vi "BAM Buffer Connections List.vi"(7 "State":T2=enum."Update", 8 "error in (no error)":errorcluster, 9 "index":i32, 10 "Connection Cluster":T3, 11 "Connections Ref":T1) -> (0 "error out":errorcluster, 1 "Connections":T3[](array[typedef]), 2 "Connection Cluster Out":T3, 3 "Connections Ref out":T1)   [LabVIEW 2015, in "J1939 Addon Engine.lvlib"]
uses:
  J1939 Addon Engine.lvlib
  Types/TP Buffer Connection Cluster.ctl
  Types/TP Connections List State.ctl
  Types/BAM Buffer Connections List_Ref.ctl
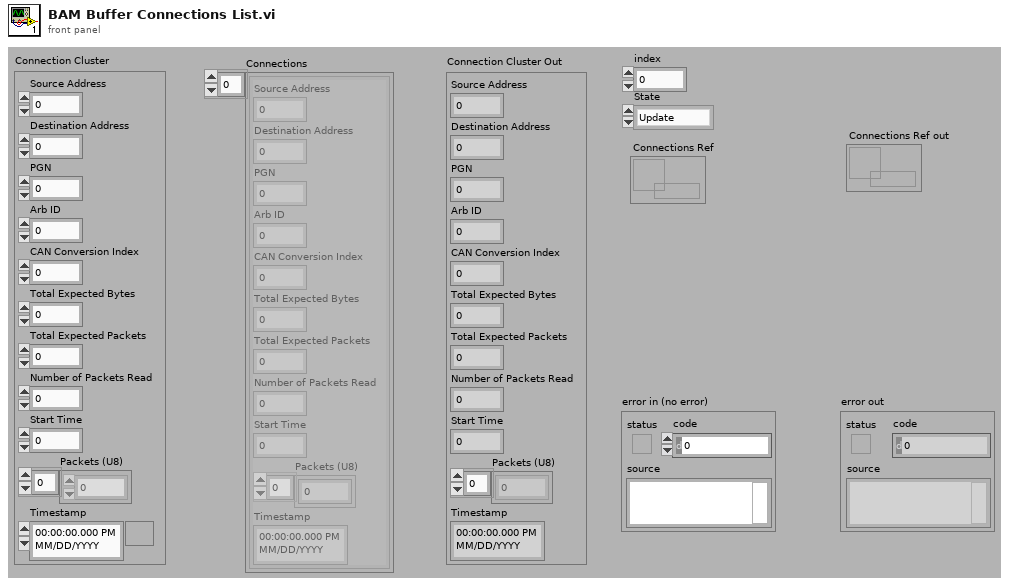
[diagram p1: front panel]
types:
  T1 = typedef "J1939 Addon Engine.lvlib/BAM Buffer Connections List_Ref.ctl" = refnum<data-value>
  T2 = typedef "J1939 Addon Engine.lvlib/TP Connections List State.ctl" = enum16{"Add", "Update", "Get", "Remove", "Initialize"}
  T3 = typedef "J1939 Addon Engine.lvlib/TP Buffer Connection Cluster.ctl" = cluster{"Source Address":u8, "Destination Address":u8, "PGN":u32, "Arb ID":u32, "CAN Conversion Index":u32, "Total Expected Bytes":u16, "Total Expected Packets":u8, "Number of Packets Read":u8, "Start Time":u32, "Packets (U8)":u8[], "Timestamp":timestamp}
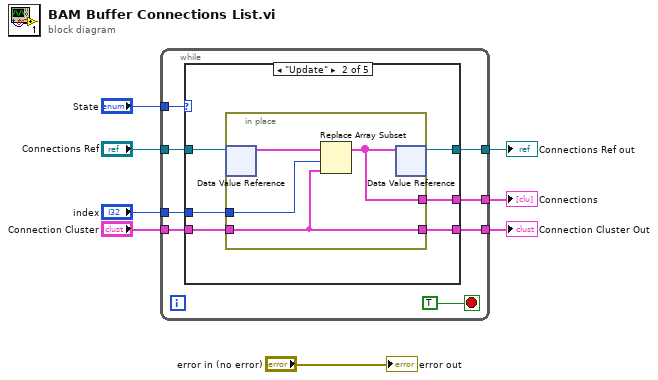
[diagram p0: block diagram]
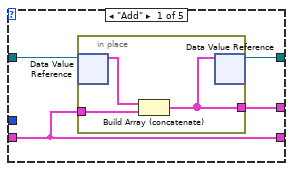
[diagram p2: hidden frame]
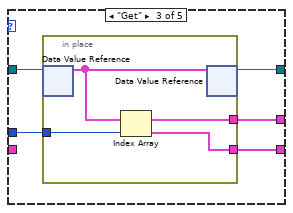
[diagram p3: hidden frame]
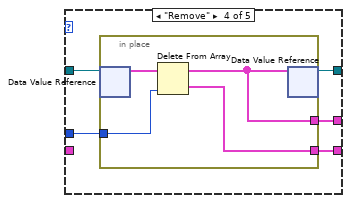
[diagram p4: hidden frame]
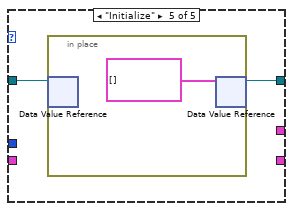
[diagram p5: hidden frame]
diagram:
  n1 = while {
    tunnel: "State" -> [w16]
    tunnel: "Connection Cluster" -> [w15]
    tunnel: "index" -> [w14]
    tunnel: [w13] -> w5
    tunnel: "Connections Ref" -> [w11]
    tunnel: [w10] -> w2
    tunnel: [w9] -> w1
    stop <- TRUE stop-if-true
    n2 = case shown="\"Update\"" w16 {
      tunnel: w15 -> [w19 w28 _ _ _]
      tunnel: [w20 w27 w34 w45 _] -> w9
      tunnel: w14 -> [_ w29 w38 w46 _]
      tunnel: [w19 w24 w37 w44 _] -> w13
      tunnel: w11 -> [w18 w26 w36 w43 w52]
      tunnel: [w17 w25 w35 w42 w51] -> w10
      frame "Add" {
        n3 = in-place {
          in-place-border: [w21] -> w20
          in-place-border: w19 -> [w23]
          n4 = in-place-dvr #1(w18) -> (w22:T3[])  [unwired: 1 out]
          n5 = Build Array (concatenate)(w22, w23) -> (w21:T3[])
          n6 = in-place-dvr #1(w21) -> (w17:T1)  [unwired: 1 out]
        }
      }
      frame "Update" {
        n7 = in-place {
          in-place-border: w29 -> [w33]
          in-place-border: w28 -> [w30]
          in-place-border: [w31] -> w27
          in-place-border: [w30] -> w24
          n8 = in-place-dvr #2(w26) -> (w32:T3[])  [unwired: 1 out]
          n9 = Replace Array Subset(array=w32, new element=w30, index=w33) -> (w31:T3[])
          n10 = in-place-dvr #2(w31) -> (w25:T1)  [unwired: 1 out]
        }
      }
      frame "Get" {
        n11 = in-place {
          in-place-border: w38 -> [w41]
          in-place-border: [w40] -> w37
          in-place-border: [w39] -> w34
          n12 = in-place-dvr #3(w36) -> (w39:T3[])  [unwired: 1 out]
          n13 = Index Array(array=w39, index=w41) -> (element=w40:T3)
          n14 = in-place-dvr #3(w39) -> (w35:T1)  [unwired: 1 out]
        }
      }
      frame "Remove" {
        n15 = in-place {
          in-place-border: w46 -> [w50]
          in-place-border: [w47] -> w45
          in-place-border: [w49] -> w44
          n16 = in-place-dvr #4(w43) -> (w48:T3[])  [unwired: 1 out]
          n17 = Delete From Array(array=w48, index=w50) -> (deleted portion=w49:T3, array with subset deleted=w47:T3[])  [unwired: 1 in]
          n18 = in-place-dvr #4(w47) -> (w42:T1)  [unwired: 1 out]
        }
      }
      frame "Initialize" {
        n19 = in-place {
          n20 = in-place-dvr #5(w52) -> ()  [unwired: 2 out]
          n21 = in-place-dvr #5(T3[] [] ("data value")) -> (w51:T1)  [unwired: 1 out]
        }
      }
    }
  }
  "Connection Cluster Out" <- w5
  "Connections" <- w1
  "Connections Ref out" <- w2
  "error out" <- "error in (no error)"
